vi "Cleanup.vi"(8 "error in (no error)":errorcluster, 11 "Barometer Bricklet in":refnum<class "Barometer Bricklet.lvclass">) -> (0 "error out":errorcluster)   [LabVIEW 2011, in "Tinkerforge.lvlib" / "Barometer Bricklet.lvclass"]
doc: "This VI is the child implementation of \"Cleanup.vi\" and releases all synchronization objects of this child object."
uses:
  Barometer Bricklet.lvclass
  Barometer Bricklet.lvclass/Barometer Bricklet.ctl
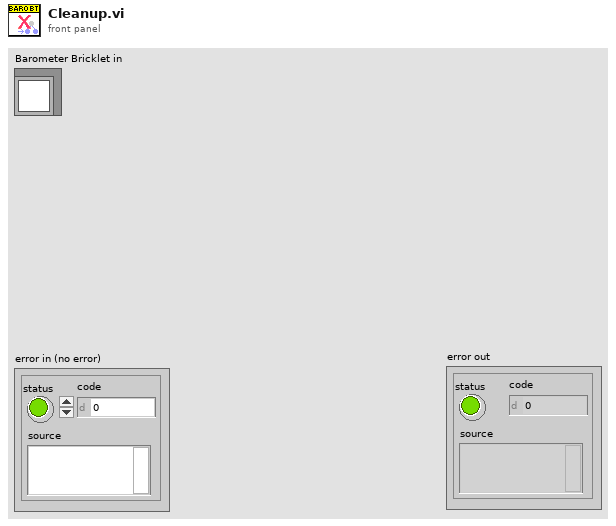
[diagram p1: front panel]
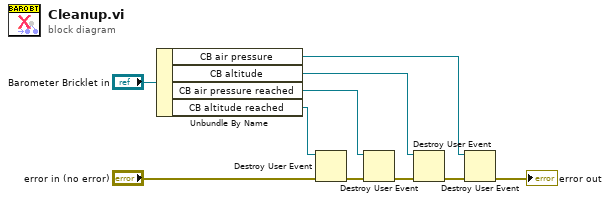
[diagram p0: block diagram]
diagram:
  n1 = Unbundle By Name("Barometer Bricklet in") -> ("CB air pressure"=w1:refnum<user-event>, "CB altitude"=w2:refnum<user-event>, "CB air pressure reached"=w3:refnum<user-event>, "CB altitude reached"=w8:refnum<user-event>)
  n2 = Destroy User Event(user event=w8, error in="error in (no error)") -> (error out=w7:errorcluster)
  n3 = Destroy User Event(user event=w3, error in=w7) -> (error out=w6:errorcluster)
  n4 = Destroy User Event(user event=w2, error in=w6) -> (error out=w5:errorcluster)
  n5 = Destroy User Event(user event=w1, error in=w5) -> (error out=→"error out":errorcluster)
